vi "dfd_Get FIR Filter Amplitude Response from TF.vi"(9 "numerator":dbl[](array[numeric]), 11 "#freq points":i32) -> (1 "Amplitude":dbl[](array[numeric]))   [LabVIEW 2017, in "NI_DigFilterLicensed.lvlib"]
uses:
  <vilib>/addons/Digital Filter Design/NI_DigFilterLicensed.lvlib
  <vilib>/Analysis/1siggen.llb/Ramp Pattern by Samples.vi
  <vilib>/Analysis/NI_AALBase.lvlib
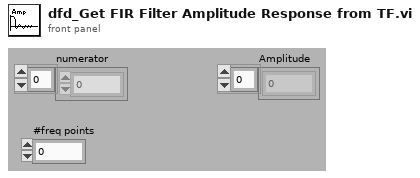
[diagram p1: front panel]
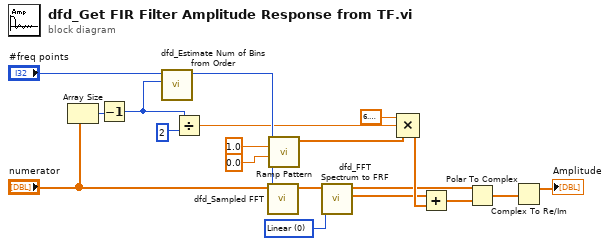
[diagram p0: block diagram]
diagram:
  w1 = u16 0 items=["Linear", "dB", "Zero phase"] ("magnitude")
  n1 = Array Size(array="numerator") -> (size(s)=w12:i32)
  n2 = Decrement(x=w12) -> (x-1=w5:i32)
  n3 = call <vilib>:"dfd_Estimate Num of Bins from Order.vi"("order"=w5, "# freq bins in"="#freq points") -> ("# freq bins out"=w4:i32)  [unwired: 9 out]
  n4 = Divide(x=w5, y=2) -> (x/y=w3:dbl)
  n5 = call <vilib>:"dfd_Sampled FFT.vi"("# freq bins (512)"=w4, "h[n]"="numerator") -> ("FFT {X}"=w10:cdb[])  [unwired: 1 in, 8 out]
  n6 = call-poly <vilib>:"Ramp Pattern.vi"("start"=0.0, "end"=1.0, "samples"=w4) -> ("Ramp Pattern"=w2:dbl[])  [unwired: 7 in, 1 out]
  n7 = call <vilib>:"dfd_FFT Spectrum to FRF.vi"("magnitude"=w1, "FFT {X}"=w10) -> ("phase"=w8:dbl[], "amplitude"=w9:dbl[])  [unwired: 3 in, 5 out]
  n8 = Compound Arithmetic op=MULTIPLY(6.283185307179586, w3, w2) -> (w15:dbl[])
  n9 = Add(x=w8, y=w15) -> (x+y=w13:dbl[])
  n10 = Polar To Complex(1:w13, 2:w9) -> (0:w16:cdb[])
  n11 = Complex To Re/Im(x + iy=w16) -> (x=→"Amplitude":dbl[])  [unwired: 1 out]
